vi "Urgent Check.vi"(4 "SR Cluster":T1 {"Creation Date" format="%<%x>T"; "Last Updated" format="%<%x>T"}) -> (0 "Past Due?":bool, 1 "Answer Today?":bool)   [LabVIEW 2018]
uses:
  Type Defs/SR Cluster.ctl
  Type Defs/SR Status.ctl
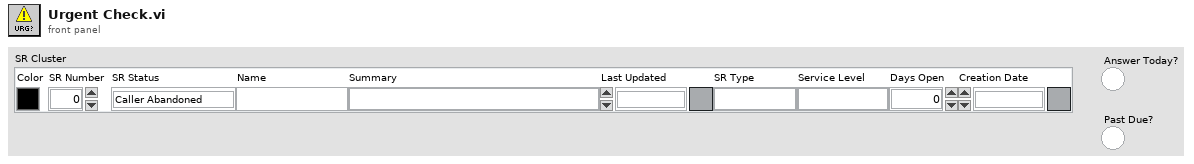
[diagram p1: front panel]
types:
  T1 = typedef "SR Cluster.ctl" = cluster{"Color":u32, "SR Number":i32, "SR Status":T2, "Name":string, "Summary":string, "Last Updated":timestamp, "SR Type":string, "Service Level":string, "Days Open":dbl, "Creation Date":timestamp}
  T2 = typedef "SR Status.ctl" = enum16{"Caller Abandoned", "Created in Error", "Expired", "Forum Resolved AE", "Forum Resolved Customer", "IN WORK", "IN WORK Collab with AES", "IN WORK Collab with PSE", "IN WORK Collab with SE", "IN WORK Customer Added Note", "IN WORK Escalation", "IN WORK Wait on Customer", "Open", "Potentially Resolved", "Presumed Resolved", "RMA Approved for Return", "RMA Closed", "RMA Closed - DOA", "RMA In Progress", "RMA Open", "RMA Waiting on Customer", "Resolved", "Passed Off"}
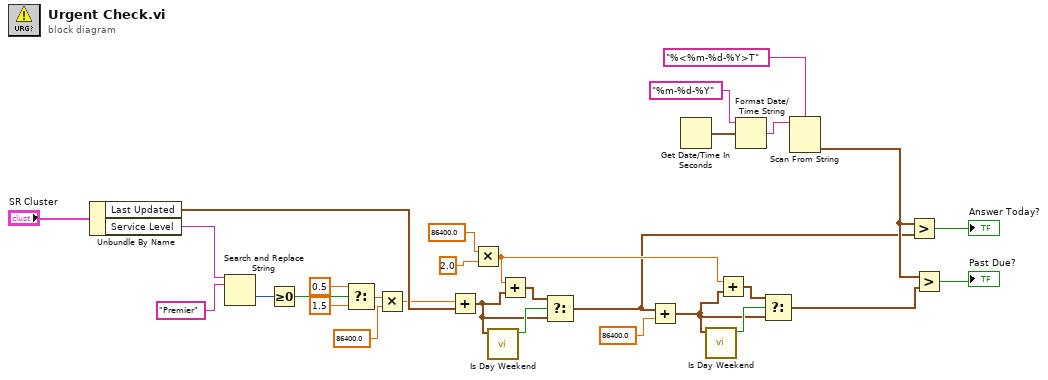
[diagram p0: block diagram]
diagram:
  n1 = Unbundle By Name("SR Cluster") -> ("Last Updated"=w12:timestamp, "Service Level"=w21:string)
  n2 = Search and Replace String(input string=w21, search string="Premier") -> (offset past replacement=w20:i32)  [unwired: 6 in, 3 out]
  n3 = Greater Or Equal To 0?(x=w20) -> (x >= 0?=w19:bool)
  n4 = Select(t=0.5, s=w19, f=1.5) -> (s? t:f=w9:dbl)
  n5 = Multiply(x=w9, y=86400.0) -> (x*y=w8:dbl)
  n6 = Add(x=w8, y=w12) -> (x+y=w16:timestamp)
  n7 = Multiply(x=86400.0 ("y"), y=2.0 ("x")) -> (x*y=w5:dbl)
  n8 = call "Is Day Weekend.vi"("Time Stamp"=w16) -> ("weekend?"=w18:bool)  [unwired: 10 in]
  n9 = Add(x=w5, y=w16) -> (x+y=w17:timestamp)
  n10 = Select(t=w17, s=w18, f=w16) -> (s? t:f=w4:timestamp)
  n11 = Add(x=w4, y=86400.0) -> (x+y=w3:timestamp)
  n12 = Get Date/Time In Seconds() -> (seconds since 1Jan1904=w24:timestamp)
  n13 = call "Is Day Weekend.vi"("Time Stamp"=w3) -> ("weekend?"=w14:bool)  [unwired: 10 in]
  n14 = Add(x=w5, y=w3) -> (x+y=w15:timestamp)
  n15 = Format Date/Time String(time format string (%c)="%m-%d-%Y" ("format string"), seconds (now)=w24) -> (date/time string=w1:string)  [unwired: 1 in]
  n16 = Select(t=w15, s=w14, f=w3) -> (s? t:f=w13:timestamp)
  n17 = Scan From String(format string="%<%m-%d-%Y>T", input string=w1) -> (output 1=w11:timestamp)  [unwired: 3 in, 3 out]
  n18 = Greater?(x=w11, y=w4) -> (0:→"Answer Today?":bool)
  n19 = Greater?(x=w11, y=w13) -> (0:→"Past Due?":bool)
